vi "create_measure_log_file.vi"(0 "Tagesordner":string) -> (7 "Messlogbuch":path)   [LabVIEW 2009]
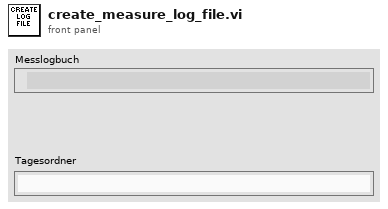
[diagram p1: front panel]
types:
  T1 = enum16{"open", "replace", "create", "open or create", "replace or create", "replace or create with confirmation"}
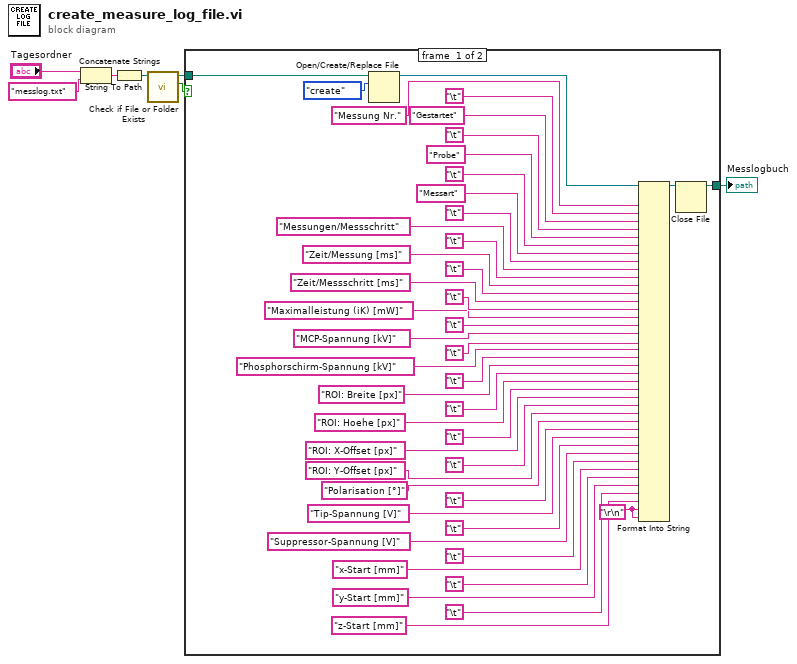
[diagram p0: block diagram]
diagram:
  n1 = Concatenate Strings("Tagesordner", "messlog.txt" ("string")) -> (w6:string)
  n2 = String To Path(string=w6) -> (path=w4:path)
  n3 = call <vilib>:"Check if File or Folder Exists.vi"("path"=w4) -> ("file or folder exists?"=w3:bool, "dup path"=w2:path)  [unwired: 8 in, 1 out]
  n4 = case shown="False" w3 {
    tunnel: w2 -> [w24 w52]
    tunnel: [w22 w52] -> w1
    frame #0 {
      w8 = "\r\n"
      n5 = Open/Create/Replace File(file path (use dialog)=w24, operation (0:open)=T1."create") -> (refnum out=w23:refnum<file>)  [unwired: 4 in, 2 out]
      n6 = Format Into String(initial string=w23, "Messung Nr." ("string"), "\t", "Gestartet" ("string"), "\t", "Probe" ("string"), "\t", "Messart" ("string"), "\t", "Messungen/Messschritt" ("string"), "\t", "Zeit/Messung [ms]" ("string"), "\t", "Zeit/Messschritt [ms]" ("string"), "\t", "Maximalleistung (iK) [mW]" ("string"), "\t", "MCP-Spannung [kV]" ("string"), "\t", "Phosphorschirm-Spannung [kV]" ("string"), "\t", "ROI: Breite [px]" ("string"), "\t", "ROI: Hoehe [px]" ("string"), "\t", "ROI: X-Offset [px]" ("string"), "\t", "ROI: Y-Offset [px]" ("string"), "Polarisation [°]" ("string"), "\t", "Tip-Spannung [V]" ("string"), "\t", "Suppressor-Spannung [V]" ("string"), "\t", "x-Start [mm]" ("string"), "\t", "y-Start [mm]" ("string"), "\t", "z-Start [mm]" ("string"), w8, w8) -> (resulting string=w25:refnum<file>)  [unwired: 2 in, 1 out]
      n7 = Close File(refnum=w25) -> (path=w22:path)  [unwired: 1 in, 1 out]
    }
    frame #1 {
    }
  }
  "Messlogbuch" <- w1
